vi "Test REF Configuration.vi"(8 "error in (no error)":errorcluster, 11 "Instrument.Lockin in":refnum<class "Instrument.Lockin.lvclass">) -> (0 "error out":errorcluster, 3 "Instrument.Lockin out":refnum<class "Instrument.Lockin.lvclass">)   [LabVIEW 2016]
uses:
  src/Instrument.Lockin/Instrument.Lockin.lvclass
  src/LockinDAQ/Typedefs/REF-cluster.ctl
  src/LockinDAQ/Typedefs/REF_Channel-Numeric.ctl
  <vilib>/addons/_JKI Toolkits/Caraya/classes/Assert/Assert Equal Value and Type_Variant.vi
  <userlib>/_OpenG.lib/numeric/numeric.llb/Random Number Within Range - DBL__ogtk.vi
  <vilib>/addons/_JKI Toolkits/Caraya/classes/Assert/Assert Almost Equal_Float.vi
  <userlib>/_OpenG.lib/numeric/numeric.llb/Random Number Within Range - I32__ogtk.vi
  <vilib>/addons/_JKI Toolkits/Caraya/classes/Test/Test.lvclass
  src/LockinDAQ/LockinDAQ.lvclass
  <vilib>/addons/_JKI Toolkits/Caraya/classes/Assert/Assert.lvclass
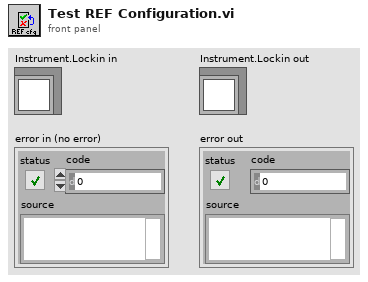
[diagram p1: front panel]
types:
  T1 = typedef "LockinDAQ.lvclass/REF-cluster.ctl" = cluster{"Ch":i32[], " f (Hz)":dbl[], "Phase (°)":dbl[], "TC (s)":dbl[], "order":i32[]}
  T2 = typedef "LockinDAQ.lvclass/REF_Channel-Numeric.ctl" = i32
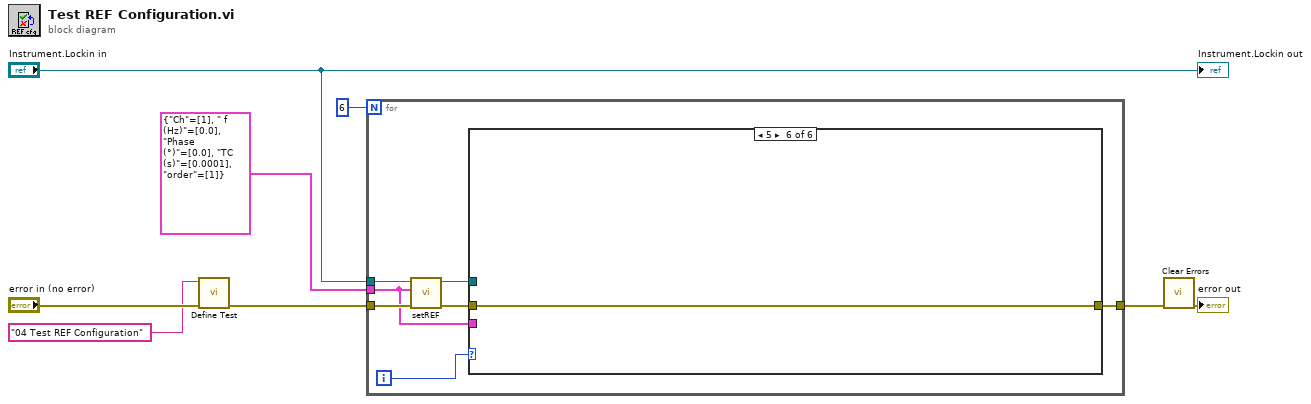
[diagram p0: block diagram]
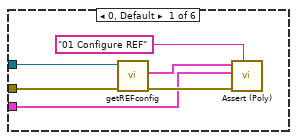
[diagram p2: hidden frame]
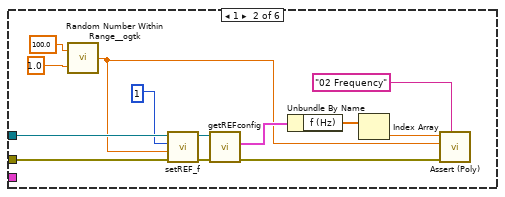
[diagram p3: hidden frame]
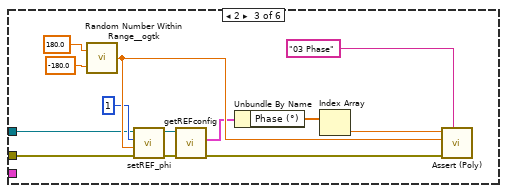
[diagram p4: hidden frame]
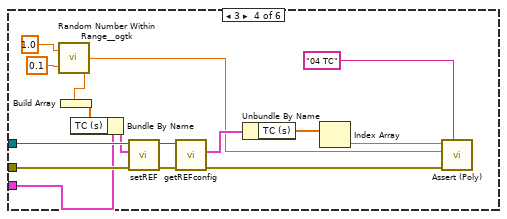
[diagram p5: hidden frame]
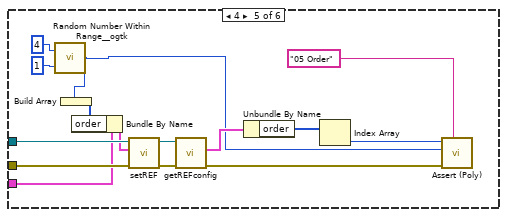
[diagram p6: hidden frame]
diagram:
  n1 = call <vilib>:"Define Test.vi"("error in (no error)"="error in (no error)", "Label (VI Title)"="04 Test REF Configuration") -> ("error out"=w4:errorcluster)  [unwired: 9 in]
  n2 = for {
    N: 6 -> [_]
    tunnel: w4 -> [w14]
    tunnel: "Instrument.Lockin in" -> [w13]
    tunnel: T1 {"Ch"=[1], " f (Hz)"=[0.0], "Phase (°)"=[0.0], "TC (s)"=[0.0001], "order"=[1]} ("Channels: Lockin in") -> [w10]
    tunnel: [w9] -> w1
    i -> [w15]
    n3 = call "setREF.vi"("error in (no error)"=w14, "Channels: Lockin in"=w10, "Instrument.Lockin in"=w13) -> ("error out"=w12:errorcluster, "Instrument.Lockin out"=w11:refnum<class "Instrument.Lockin.lvclass">)  [unwired: 7 in]
    n4 = case shown="5" w15 {
      tunnel: w12 -> [w18 w25 w36 w52 w69 w78]
      tunnel: w11 -> [w17 w24 w35 w53 w70 _]
      tunnel: w10 -> [w16 _ _ w51 w63 _]
      tunnel: [_ _ _ _ _ w78] -> w9
      frame 0, Default {
        n5 = call "getREFconfig.vi"("error in (no error)"=w18, "Instrument.Lockin in"=w17) -> ("error out"=w20:errorcluster, "REFconfig"=w19:T1)  [unwired: 7 in, 1 out]
        n6 = call-poly <vilib>:"Assert (Poly).vi"("Label"="01 Configure REF", "error in (no error)"=w20, "Y"=w16, "X"=w19) -> ()  [unwired: 7 in, 1 out]
      }
      frame 1 {
        n7 = call-poly <userlib>:"Random Number Within Range__ogtk.vi"("High"=100.0, "Low"=1.0) -> ("Random Number"=w22:dbl)  [unwired: 3 in]
        n8 = call "setREF_f.vi"("error in (no error)"=w25, "Frequency (Hz)"=w22, "REF Channel"=T2 1, "Instrument.Lockin in"=w24) -> ("error out"=w26:errorcluster, "Instrument.Lockin out"=w27:refnum<class "Instrument.Lockin.lvclass">)  [unwired: 6 in]
        n9 = call "getREFconfig.vi"("error in (no error)"=w26, "Instrument.Lockin in"=w27) -> ("error out"=w30:errorcluster, "REFconfig"=w31:T1)  [unwired: 7 in, 1 out]
        n10 = Unbundle By Name(w31) -> ("f (Hz)"=w32:dbl[])
        n11 = Index Array(array=w32) -> (element=w33:dbl)  [unwired: 1 in]
        n12 = call-poly <vilib>:"Assert (Poly).vi"("Label"="02 Frequency", "error in (no error)"=w30, "Y"=w22, "X"=w33) -> ()  [unwired: 7 in, 1 out]
      }
      frame 2 {
        n13 = call-poly <userlib>:"Random Number Within Range__ogtk.vi"("High"=180.0, "Low"=-180.0) -> ("Random Number"=w45:dbl)  [unwired: 3 in]
        n14 = call "setREF_phi.vi"("error in (no error)"=w36, "Phase (°)"=w45, "REF Channel"=T2 1, "Instrument.Lockin in"=w35) -> ("error out"=w37:errorcluster, "Instrument.Lockin out"=w38:refnum<class "Instrument.Lockin.lvclass">)  [unwired: 6 in]
        n15 = call "getREFconfig.vi"("error in (no error)"=w37, "Instrument.Lockin in"=w38) -> ("error out"=w46:errorcluster, "REFconfig"=w43:T1)  [unwired: 7 in, 1 out]
        n16 = Unbundle By Name(w43) -> ("Phase (°)"=w42:dbl[])
        n17 = Index Array(array=w42) -> (element=w44:dbl)  [unwired: 1 in]
        n18 = call-poly <vilib>:"Assert (Poly).vi"("Label"="03 Phase", "error in (no error)"=w46, "Y"=w45, "X"=w44) -> ()  [unwired: 7 in, 1 out]
      }
      frame 3 {
        n19 = call-poly <userlib>:"Random Number Within Range__ogtk.vi"("High"=1.0, "Low"=0.1) -> ("Random Number"=w49:dbl)  [unwired: 3 in]
        n20 = Build Array(w49) -> (w48:dbl[])
        n21 = Bundle By Name(cluster=w51, "TC (s)"=w48) -> (w50:T1)
        n22 = call "setREF.vi"("error in (no error)"=w52, "Channels: Lockin in"=w50, "Instrument.Lockin in"=w53) -> ("error out"=w55:errorcluster, "Instrument.Lockin out"=w54:refnum<class "Instrument.Lockin.lvclass">)  [unwired: 7 in]
        n23 = call "getREFconfig.vi"("error in (no error)"=w55, "Instrument.Lockin in"=w54) -> ("error out"=w61:errorcluster, "REFconfig"=w59:T1)  [unwired: 7 in, 1 out]
        n24 = Unbundle By Name(w59) -> ("TC (s)"=w58:dbl[])
        n25 = Index Array(array=w58) -> (element=w60:dbl)  [unwired: 1 in]
        n26 = call-poly <vilib>:"Assert (Poly).vi"("Label"="04 TC", "error in (no error)"=w61, "Y"=w49, "X"=w60) -> ()  [unwired: 7 in, 1 out]
      }
      frame 4 {
        n27 = call-poly <userlib>:"Random Number Within Range__ogtk.vi"("High"=4, "Low"=1) -> ("Random Number"=w64:i32)  [unwired: 3 in]
        n28 = Build Array(w64) -> (w67:i32[])
        n29 = Bundle By Name(cluster=w63, "order"=w67) -> (w68:T1)
        n30 = call "setREF.vi"("error in (no error)"=w69, "Channels: Lockin in"=w68, "Instrument.Lockin in"=w70) -> ("error out"=w72:errorcluster, "Instrument.Lockin out"=w71:refnum<class "Instrument.Lockin.lvclass">)  [unwired: 7 in]
        n31 = call "getREFconfig.vi"("error in (no error)"=w72, "Instrument.Lockin in"=w71) -> ("error out"=w76:errorcluster, "REFconfig"=w74:T1)  [unwired: 7 in, 1 out]
        n32 = Unbundle By Name(w74) -> ("order"=w73:i32[])
        n33 = Index Array(array=w73) -> (element=w75:i32)  [unwired: 1 in]
        n34 = call-poly <vilib>:"Assert (Poly).vi"("Label"="05 Order", "error in (no error)"=w76, "Y"=w64, "X"=w75) -> ()  [unwired: 7 in, 1 out]
      }
      frame 5 {
      }
    }
  }
  n35 = call <vilib>:"Clear Errors.vi"("error in (no error)"=w1) -> ("error out"=→"error out":errorcluster)  [unwired: 5 in, 1 out]
  "Instrument.Lockin out" <- "Instrument.Lockin in"
